vi "Write Service Name.vi"(10 "Service Name":string, 11 "UDP Service in":refnum<class "UDP Service.lvclass">) -> (3 "UDP Service out":refnum<class "UDP Service.lvclass">)   [LabVIEW 2016, in "UDP Service.lvlib" / "UDP Service.lvclass"]
uses:
  UDP Service.lvclass
  UDP Service.lvclass/UDP Service.ctl
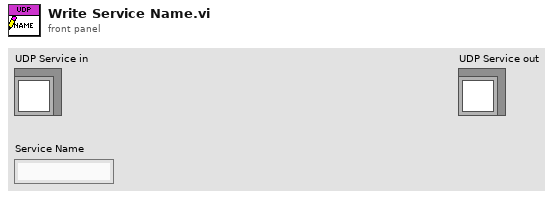
[diagram p1: front panel]
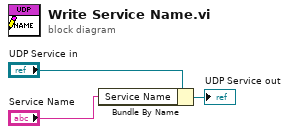
[diagram p0: block diagram]
diagram:
  n1 = Bundle By Name(cluster="UDP Service in", "Service Name"="Service Name") -> (→"UDP Service out":refnum<class "UDP Service.lvclass">)
